vi "Init.vi"(8 "error in (no error)":errorcluster, 10 "Enqueuer":refnum<class "Message Enqueuer.lvclass">) -> (0 "error out":errorcluster, 3 "VMR Actor API out":refnum<class "VMR Actor API.lvclass">)   [LabVIEW 2022 SP3, in "VMR Server.lvlib" / "VMR Actor API.lvclass"]
uses:
  VMR Actor API.lvclass
  VMR Actor API.lvclass/VMR Actor API.ctl
  <vilib>/ActorFramework/Message Enqueuer/Message Enqueuer.lvclass
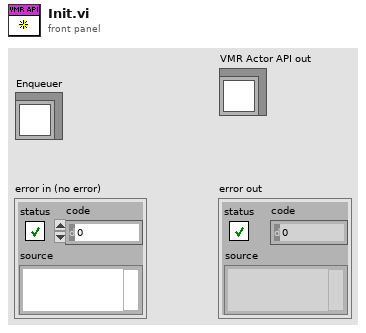
[diagram p1: front panel]
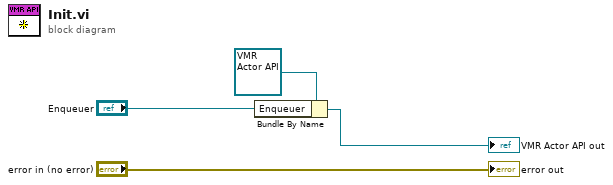
[diagram p0: block diagram]
diagram:
  n1 = Bundle By Name(cluster=refnum<class "VMR Actor API.lvclass"> refnum ("VMR Actor API in"), "Enqueuer"="Enqueuer") -> (→"VMR Actor API out":refnum<class "VMR Actor API.lvclass">)
  "error out" <- "error in (no error)"
